vi "Throw JSON Error - Parse Error.vi"(8 "error in (no error)":errorcluster, 9 "additional info":string, 11 "datatype":string) -> (0 "error out":errorcluster)   [LabVIEW 2014, in "i3-json.lvlib"]
uses:
  i3-json.lvlib
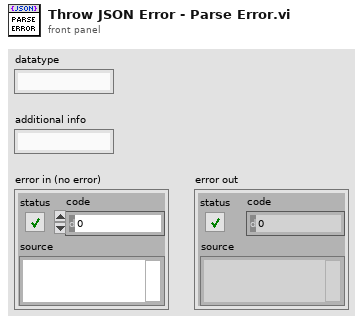
[diagram p1: front panel]
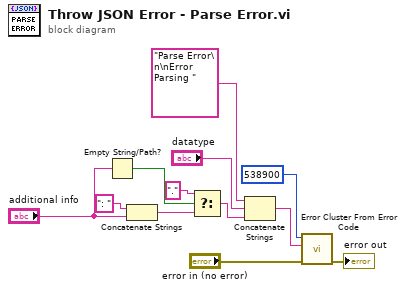
[diagram p0: block diagram]
diagram:
  n1 = Empty String/Path?(string/path="additional info") -> (empty?=w9:bool)
  n2 = Concatenate Strings(": " ("string"), "additional info") -> (w1:string)
  n3 = Select(t="." ("datatype"), s=w9, f=w1) -> (s? t:f=w7:string)
  n4 = Concatenate Strings("Parse Error\n\nError Parsing " ("error message (\"\")"), "datatype", w7) -> (w6:string)
  n5 = call <vilib>:"Error Cluster From Error Code.vi"("error in (no error)"="error in (no error)", "error message (\"\")"=w6, "error code (0)"=538900) -> ("error out"=→"error out":errorcluster)  [unwired: 6 in]
